vi "setMethods.vi"(0 "reference":refnum<class "ClassNode.lvclass">, 1 "name":refnum<class "MultiLineString.lvclass">, 5 "error in (no error)":errorcluster) -> (14 "reference out":refnum<class "ClassNode.lvclass">, 19 "error out":errorcluster)   [LabVIEW 2012, in "ClassNode.lvclass"]
doc: "public void setMethods(MultiLineString newValue)"
uses:
  <resource>/Framework/Providers/Open_GDS/UML/ClassNode_class/ClassNode.lvclass
  <resource>/Framework/Providers/Open_GDS/UML/MultiLineString_class/MultiLineString.lvclass
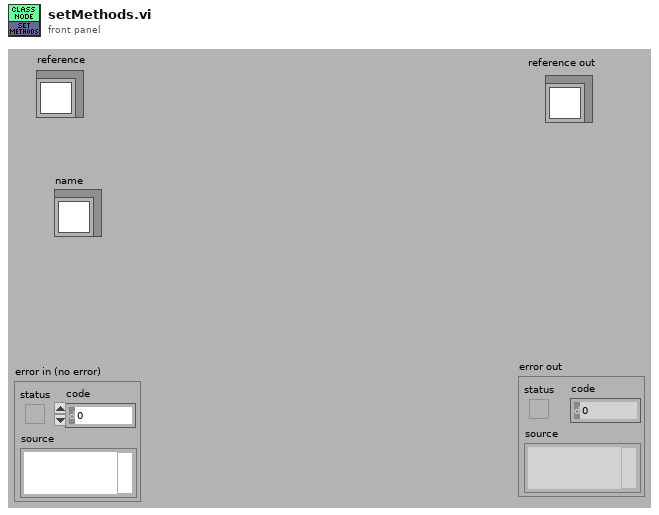
[diagram p1: front panel]
types:
  T1 = typedef "ClassNode.lvclass/ObjectAttributes.ctl" = cluster{"Base class":T2, "midHeight":dbl, "botHeight":dbl, "name":refnum<class "MultiLineString.lvclass">, "attributes":refnum<class "MultiLineString.lvclass">, "methods":refnum<class "MultiLineString.lvclass">, "DEFAULT_COMPARTMENT_HEIGHT":i32, "DEFAULT_WIDTH":i32, "DEFAULT_HEIGHT":i32, "showMethods":bool, "showAttributes":bool, "ClassPath":path}
  T2 = typedef "RectangularNode.lvclass/ObjectAttributes.ctl" = cluster{"Base class":T3, "bounds":T4}
  T3 = typedef "AbstractNode.lvclass/ObjectAttributes.ctl" = cluster{"parent":refnum<class "AbstractNode.lvclass">, "children":refnum<class "AbstractNode.lvclass">[], "Hidden":bool}
  T4 = typedef "Rectangle Rectangle2D.ctl" = cluster{"x":dbl, "y":dbl, "width":dbl, "height":dbl}
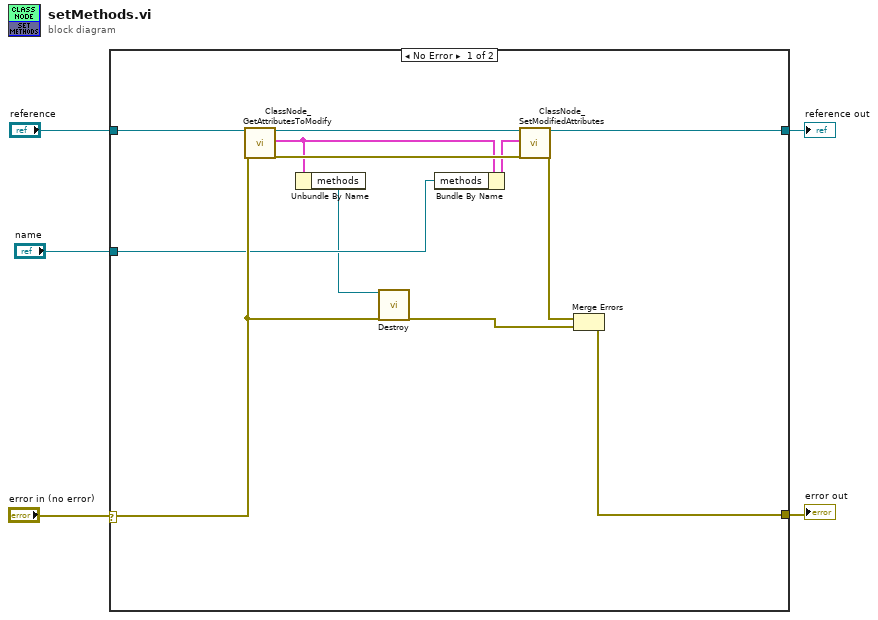
[diagram p0: block diagram]
diagram:
  n1 = case shown="No Error" "error in (no error)" {
    selector: "error in (no error)" -> [w14 w18]
    tunnel: "reference" -> [w17 w19]
    tunnel: [w16 w18] -> w4
    tunnel: [w15 w19] -> w3
    tunnel: "name" -> [w13 _]
    frame No Error {
      n2 = call <resource>:"ClassNode_GetAttributesToModify.vi"("reference in"=w17, "error in (no error)"=w14) -> ("reference out"=w11:refnum<class "ClassNode.lvclass">, "Attributes"=w10:T1, "error out"=w12:errorcluster)  [unwired: 1 in, 14 out]
      n3 = Unbundle By Name(w10) -> ("methods"=w8:refnum<class "MultiLineString.lvclass">)
      n4 = call-dynamic "Destroy.vi"("reference"=w8, "error in (no error)"=w14) -> ("error out"=w7:errorcluster)  [unwired: 17 out]
      n5 = Bundle By Name(cluster=w10, "methods"=w13) -> (w9:T1)
      n6 = call <resource>:"ClassNode_SetModifiedAttributes.vi"("reference in"=w11, "Attributes"=w9, "error in (no error)"=w12) -> ("reference out"=w15:refnum<class "ClassNode.lvclass">, "error out"=w6:errorcluster)  [unwired: 3 in, 12 out]
      n7 = Merge Errors(w6, w7) -> (w16:errorcluster)
    }
    frame Error {
    }
  }
  "reference out" <- w3
  "error out" <- w4
